vi "SVL Scale Voltage to EU (1 Ch).vi"(7 "write waveform attributes? (T)":bool=TRUE, 8 "error in (no error)":errorcluster, 10 "channel info":T1={"sensor sensitivity"=1000.0, "engineering units"=1, "dB reference"=1.0, "custom label"="EU", "weighting filter"=0, "pregain"=0.0} {"pregain" format="%.2f"; "weighting filter" items=["Linear", "A-weighting", "B-weighting", "C-weighting", "ITU-R 468-4", "Dolby", "CCITT", "C-message", "Wb", "Wc", "Wd", "We", "Wf", "Wh", "Wj", "Wk", "Wm", "AES17 20 kHz lowpass", "AES17 40 kHz lowpass", "AES17 20 kHz highpass", "AES17 40 kHz highpass"]; "dB reference" format="%^.1e"; "engineering units" items=["custom..."=0, "V"=1, "A"=21, "C"=30, "pC"=31, "s"=32, "-"=29, "Pa"=2, "N"=20, "g"=3, "m/s^2"=4, "m/s"=5, "m"=6, "mm/s"=12, "mm"=13, "micron/s"=14, "micron"=15, "in/s^2"=7, "in/s"=8, "in"=9, "mil/s"=10, "mil"=11, "rad/s^2"=16, "rad/s"=17, "rad"=18, "deg/s^2"=26, "deg/s"=27, "deg"=28, "RPM"=22, "cycle/s^2"=23, "Hz"=24, "cycle"=25, "strain"=19]; "sensor sensitivity" format="%#_5f"}, 11 "signal [V]":waveform(dbl)={"t0"=timestamp(0 s since 1904-01-01), "dt"=0.0, "Y"=[]}) -> (0 "error out":errorcluster, 2 "unit label":string, 3 "scaled signal [EU]":waveform(dbl))   [LabVIEW 2017, in "SoundVib_Calibration.lvlib"]
doc: "Scales <B>signal [V]</B> from volts to the engineering units (EU) you select. Wire data to the <B>signal [V]</B> input to determine the polymorphic instance to use or manually select the instance."
uses:
  <vilib>/addons/Sound and Vibration/svt_Calibration/SoundVib_Calibration.lvlib
  <vilib>/addons/_NISVFA/_Shared subVIs/Controls/svc_Channel Info.ctl
  <vilib>/addons/_NISVFA/_Shared subVIs/Controls/svc_Engineering Units Text Ring.ctl
  <vilib>/addons/_NISVFA/_Shared subVIs/Controls/svc_Weighting Filter Text Ring.ctl
  <vilib>/addons/_NISVFA/_Shared subVIs/Common/svc_Set SV Channel Info (variant).vi
  <vilib>/addons/_NISVFA/_Shared subVIs/Common/SVL Set dB Reference (variant).vi
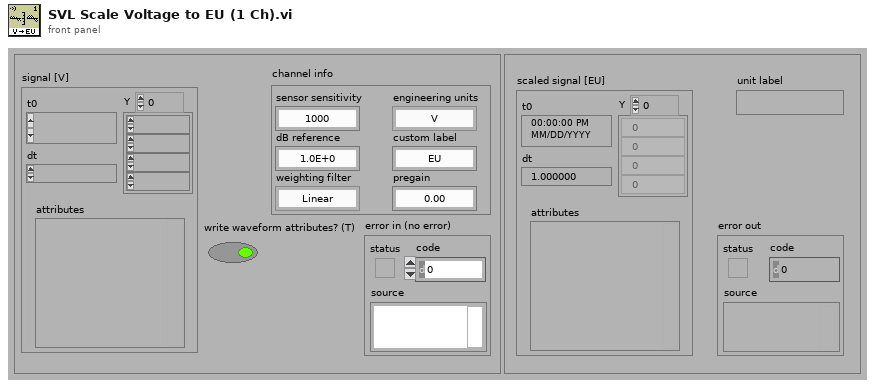
[diagram p1: front panel]
types:
  T1 = typedef "svc_Channel Info.ctl" = cluster{"sensor sensitivity":dbl, "engineering units":T2, "dB reference":dbl, "custom label":string, "weighting filter":T3, "pregain":dbl}
  T2 = typedef "svc_Engineering Units Text Ring.ctl" = u16
  T3 = typedef "svc_Weighting Filter Text Ring.ctl" = u16
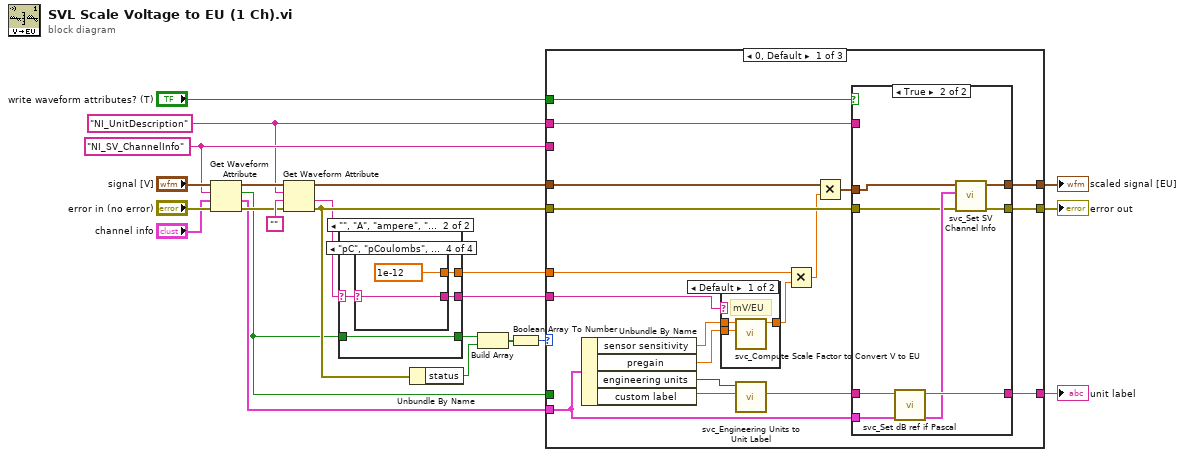
[diagram p0: block diagram]
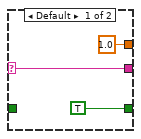
[diagram p2: hidden frame]
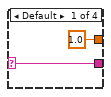
[diagram p3: hidden frame]
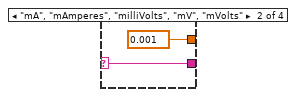
[diagram p4: hidden frame]
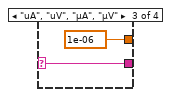
[diagram p5: hidden frame]
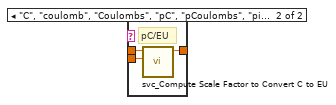
[diagram p6: hidden frame]
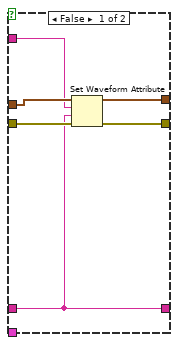
[diagram p7: hidden frame]
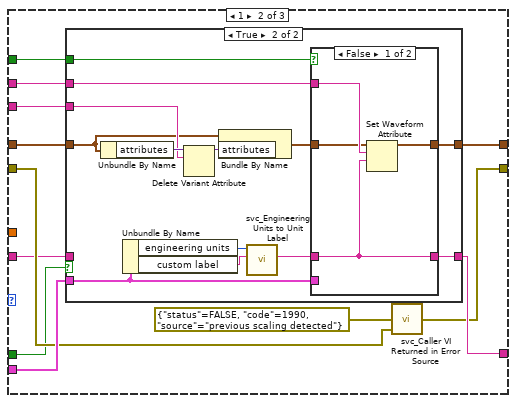
[diagram p8: hidden frame]
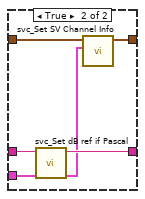
[diagram p10: hidden frame]
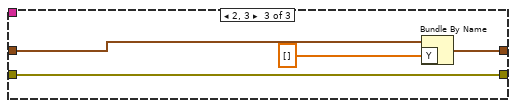
[diagram p11: hidden frame]
diagram:
  w4 = "NI_UnitDescription" ("name")
  w17 = "NI_SV_ChannelInfo" ("name")
  n1 = Get Waveform Attribute(4:"error in (no error)", 5:"channel info", 6:w17, 7:"signal [V]") -> (0:w14:errorcluster, 1:w12:T1, 2:w6:bool, 3:w13:waveform(dbl))
  n2 = Get Waveform Attribute(4:w14, 5:"", 6:w4, 7:w13) -> (0:w11:errorcluster, 1:w2:string, 3:w16:waveform(dbl))  [unwired: 1 out]
  n3 = case shown="\"\", \"A\", \"ampere\", \"Amperes\", \"C\", \"coulomb\", \"Coulombs\", \"mA\", \"mV\", \"pC\", \"pCoulombs\", \"picoCoulombs\", \"uA\", \"uV\", \"V\", \"volt\", \"Volts\", \"µA\", \"µV\"" w2 {
    selector: w2 -> [w24 w29]
    tunnel: w6 -> [_ w30]
    tunnel: [TRUE w30] -> w9
    tunnel: [1.0 ("y") w28] -> w3
    tunnel: [w24 w27] -> w1
    frame Default {
    }
    frame "", "A", "ampere", "Amperes", "C", "coulomb", "Coulombs", "mA", "mV", "pC", "pCoulombs", "picoCoulombs", "uA", "uV", "V", "volt", "Volts", "µA", "µV" {
      n4 = case shown="\"pC\", \"pCoulombs\", \"picoCoulombs\"" w29 {
        selector: w29 -> [w31 w33 w35 w37]
        tunnel: [1.0 ("y") 0.001 ("y") 1e-06 ("y") 1e-12 ("y")] -> w28
        tunnel: [w31 w33 w35 w37] -> w27
        frame Default {
        }
        frame "mA", "mAmperes", "milliVolts", "mV", "mVolts" {
        }
        frame "uA", "uV", "µA", "µV" {
        }
        frame "pC", "pCoulombs", "picoCoulombs" {
        }
      }
    }
  }
  n5 = Unbundle By Name(w11) -> ("status"=w10:bool)
  n6 = Build Array(w9, w10) -> (w8:bool[])
  n7 = Boolean Array To Number(Boolean array=w8) -> (number=w7:u32)
  n8 = case shown="0, Default" w7 {
    tunnel: [w54 w79 w115] -> w22
    tunnel: w11 -> [w45 w86 w114]
    tunnel: [w56 w88 _] -> w19
    tunnel: [w53 w84 w114] -> w21
    tunnel: w12 -> [w46 w87 _]
    tunnel: w16 -> [w52 w81 w117]
    tunnel: w1 -> [w39 w82 _]
    tunnel: w6 -> [_ w83 _]
    tunnel: w17 -> [_ w80 _]
    tunnel: "write waveform attributes? (T)" -> [w44 w78 _]
    tunnel: w4 -> [w43 w77 _]
    tunnel: w3 -> [w42 _ _]
    frame 0, Default {
      n9 = Unbundle By Name(w46) -> ("sensor sensitivity"=w51:dbl, "pregain"=w50:dbl, "engineering units"=w49:T2, "custom label"=w48:string)
      n10 = case shown="Default" w39 {
        tunnel: w51 -> [w59 w62]
        tunnel: w50 -> [w58 w61]
        tunnel: [w57 w60] -> w41
        frame Default {
          # "mV/EU"
          n11 = call <vilib>:"svc_Compute Scale Factor to Convert V to EU.vi"("pregain [dB]"=w58, "sensor sensitivity [mV/EU]"=w59) -> ("EU scale factor [EU/V]"=w57:dbl)  [unwired: 9 in]
        }
        frame "C", "coulomb", "Coulombs", "pC", "pCoulombs", "picoCoulombs" {
          # "pC/EU"
          n12 = call <vilib>:"svc_Compute Scale Factor to Convert C to EU.vi"("pregain [dB]"=w61, "sensor sensitivity [pC/EU]"=w62) -> ("EU scale factor [EU/C]"=w60:dbl)  [unwired: 9 in]
        }
      }
      n13 = call <vilib>:"svc_Engineering Units to Unit Label.vi"("custom label"=w48, "engineering units"=w49) -> ("unit label"=w47:string)  [unwired: 8 in, 1 out]
      n14 = Multiply(x=w42, y=w41) -> (x*y=w40:dbl)
      n15 = Multiply(x=w52, y=w40) -> (x*y=w55:waveform(dbl))
      n16 = case shown="True" w44 {
        tunnel: [w67 w76] -> w56
        tunnel: w55 -> [w65 w75]
        tunnel: [w63 w74] -> w54
        tunnel: [w66 w73] -> w53
        tunnel: w47 -> [w67 w71]
        tunnel: w46 -> [_ w70]
        tunnel: w45 -> [w68 w69]
        tunnel: w43 -> [w64 _]
        frame False {
          n17 = Set Waveform Attribute(4:w68, 5:w67, 6:w64, 7:w65) -> (0:w66:errorcluster, 3:w63:waveform(dbl))  [unwired: 1 out]
        }
        frame True {
          n18 = call <vilib>:"svc_Set dB ref if Pascal.vi"("channel info"=w70, "unit label"=w71) -> ("channel info"=w72:T1, "dup unit label"=w76:string)  [unwired: 4 in]
          n19 = call <vilib>:"svc_Set SV Channel Info.vi"("error in (no error)"=w69, "channel info"=w72, "scaled signal in"=w75) -> ("error out"=w73:errorcluster, "scaled signal out"=w74:waveform(dbl))  [unwired: 7 in]
        }
      }
    }
    frame 1 {
      n20 = case shown="True" w83 {
        tunnel: [w89 w100] -> w88
        tunnel: w87 -> [_ w99]
        tunnel: w82 -> [w89 _]
        tunnel: w81 -> [w90 w93]
        tunnel: w80 -> [_ w97]
        tunnel: [w90 w94] -> w79
        tunnel: w78 -> [_ w92]
        tunnel: w77 -> [_ w91]
        frame False {
        }
        frame True {
          n21 = Unbundle By Name(w93) -> ("attributes"=w98:variant)
          n22 = Unbundle By Name(w99) -> ("engineering units"=w103:T2, "custom label"=w102:string)
          n23 = Delete Variant Attribute(6:w97, 7:w98) -> (3:w96:variant)  [unwired: 1 in, 2 out]
          n24 = Bundle By Name(cluster=w93, "attributes"=w96) -> (w95:waveform(dbl))
          n25 = call <vilib>:"svc_Engineering Units to Unit Label.vi"("custom label"=w102, "engineering units"=w103) -> ("unit label"=w101:string)  [unwired: 8 in, 1 out]
          n26 = case shown="False" w92 {
            tunnel: w101 -> [w107 w113]
            tunnel: [w107 w112] -> w100
            tunnel: w99 -> [_ w111]
            tunnel: w95 -> [w104 w110]
            tunnel: [w105 w108] -> w94
            tunnel: w91 -> [w106 _]
            frame False {
              n27 = Set Waveform Attribute(5:w107, 6:w106, 7:w104) -> (3:w105:waveform(dbl))  [unwired: 1 in, 2 out]
            }
            frame True {
              n28 = call <vilib>:"svc_Set dB ref if Pascal.vi"("channel info"=w111, "unit label"=w113) -> ("channel info"=w109:T1, "dup unit label"=w112:string)  [unwired: 4 in]
              n29 = call <vilib>:"svc_Set SV Channel Info.vi"("channel info"=w109, "scaled signal in"=w110) -> ("scaled signal out"=w108:waveform(dbl))  [unwired: 8 in, 1 out]
            }
          }
        }
      }
      n30 = call <vilib>:"svc_Caller VI Returned in Error Source.vi"("warning input to caller"=w86, "error in (no error)"=errorcluster {"status"=FALSE, "code"=1990, "source"="previous scaling detected"} ("error out")) -> ("error out"=w84:errorcluster)  [unwired: 3 in]
    }
    frame 2, 3 {
      n31 = Bundle By Name(cluster=w117, "Y"=dbl[] []) -> (w115:waveform(dbl))
    }
  }
  "scaled signal [EU]" <- w22
  "error out" <- w21
  "unit label" <- w19
